vi "Cryomagnetics Get Controls.vi"(8 "error in (no error)":errorcluster, 10 "Data in":T1 {"Fast rate" format="%.4g"; "Low limit, kG" format="%.3g"; "High limit, kG" format="%.3g"; "Rates, A/s" format="%.4g"}, 11 "VISA resource name":refnum<visa-resource-name>) -> (0 "error out":errorcluster, 2 "Data out":T1 {"Fast rate" format="%.4g"; "Low limit, kG" format="%.3g"; "High limit, kG" format="%.3g"; "Rates, A/s" format="%.4g"}, 3 "VISA Resource Name Out":refnum<visa-resource-name>)   [LabVIEW 2015]
uses:
  Cryomagnetics Control Panel Data.ctl
  Sweep mode.ctl
  GPIB/VISA  Send Receive.vi
panel:
  out "Low limit, kG":dbl format="%.3g"
  out "High limit, kG":dbl format="%.3g"
  out "Fast rate":dbl format="%.4g"
  out "Rates":dbl[](array[numeric]) format="%.4g"
  out "Ranges":dbl[](array[numeric])
  # "Magnet Control"
  # "Magnet Control"
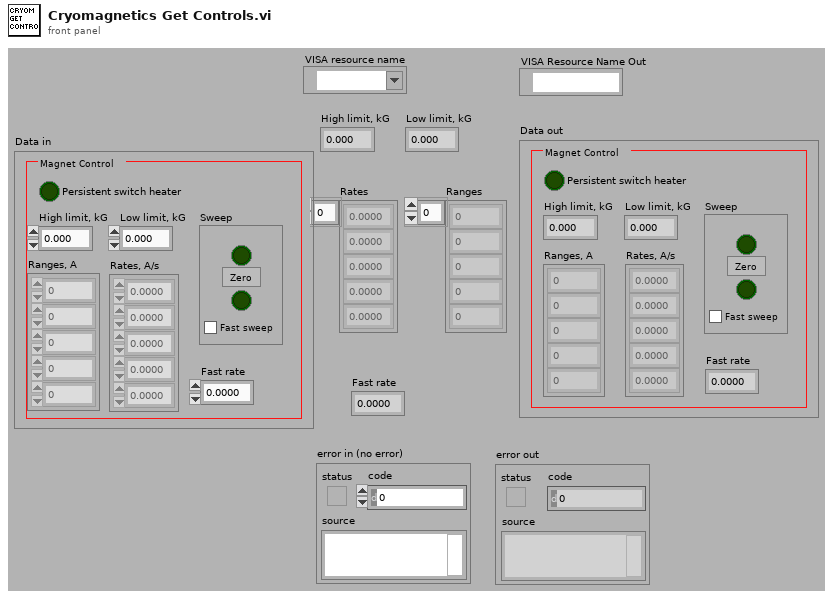
[diagram p1: front panel]
types:
  T1 = typedef "Cryomagnetics Control Panel Data.ctl" = cluster{"Persistent switch heater":bool, "Rates, A/s":dbl[], "Ranges, A":dbl[], "High limit, kG":dbl, "Low limit, kG":dbl, "Sweep ":T2, "Fast rate":dbl}
  T2 = typedef "Sweep mode.ctl" = cluster{"zero":bool, "sweep up":bool, "sweep down":bool, "fast sweep":bool}
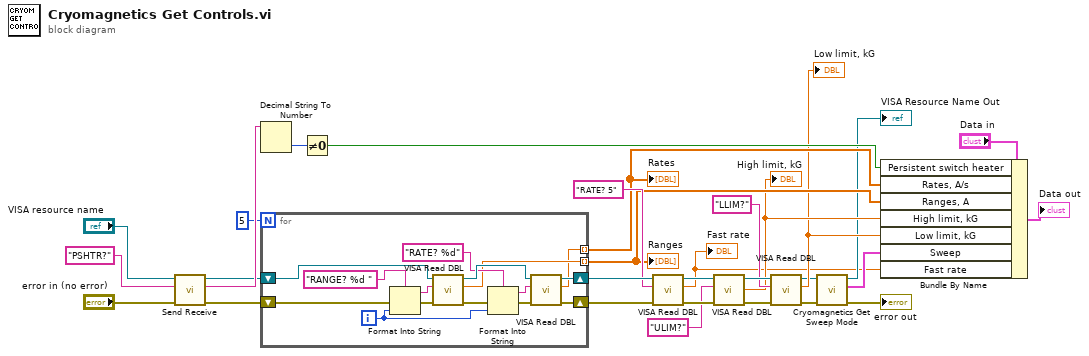
[diagram p0: block diagram]
diagram:
  n1 = call-poly "Send Receive.vi"("error in (no error)"="error in (no error)", "data string in"="PSHTR?", "VISA Resource Name"="VISA resource name") -> ("error out"=w6:errorcluster, "data string out"=w27:string, "VISA Resource Name Out"=w5:refnum<visa-resource-name>)  [unwired: 6 in]
  n2 = Decimal String To Number(string=w27) -> (number=w26:i32)  [unwired: 2 in, 1 out]
  n3 = for {
    N: 5 -> [_]
    shift-right: [w39] -> w23
    shift-left: w5 -> [w45]
    shift-right: [w33] -> w24
    shift-left: w6 -> [w42]
    tunnel: [w32] -> w12 mode=indexing
    tunnel: [w31] -> w13 mode=indexing
    i -> [w37]
    n4 = Format Into String(format string="RANGE? %d ", error in=w42, w37) -> (resulting string=w43:string, error out=w41:errorcluster)  [unwired: 1 in]
    n5 = call "VISA Read DBL.vi"("error in"=w41, "Query string"=w43, "VISA Resource Name"=w45) -> ("error out"=w36:errorcluster, "Value"=w32:dbl, "VISA Resource Name Out"=w40:refnum<visa-resource-name>)  [unwired: 6 in]
    n6 = Format Into String(format string="RATE? %d", error in=w36, w37) -> (resulting string=w34:string, error out=w35:errorcluster)  [unwired: 1 in]
    n7 = call "VISA Read DBL.vi"("error in"=w35, "Query string"=w34, "VISA Resource Name"=w40) -> ("error out"=w33:errorcluster, "Value"=w31:dbl, "VISA Resource Name Out"=w39:refnum<visa-resource-name>)  [unwired: 6 in]
  }
  "Ranges" <- w12
  "Rates" <- w13
  n8 = Not Equal To 0?(x=w26) -> (x != 0?=w14:bool)
  n9 = call "VISA Read DBL.vi"("error in"=w24, "Query string"="RATE? 5" ("data string in"), "VISA Resource Name"=w23) -> ("error out"=w21:errorcluster, "Value"=w2:dbl, "VISA Resource Name Out"=w20:refnum<visa-resource-name>)  [unwired: 6 in]
  "Fast rate" <- w2
  n10 = call "VISA Read DBL.vi"("error in"=w21, "Query string"="ULIM?" ("data string in"), "VISA Resource Name"=w20) -> ("error out"=w18:errorcluster, "Value"=w11:dbl, "VISA Resource Name Out"=w17:refnum<visa-resource-name>)  [unwired: 6 in]
  "High limit, kG" <- w11
  n11 = call "VISA Read DBL.vi"("error in"=w18, "Query string"="LLIM?" ("data string in"), "VISA Resource Name"=w17) -> ("error out"=w9:errorcluster, "Value"=w10:dbl, "VISA Resource Name Out"=w8:refnum<visa-resource-name>)  [unwired: 6 in]
  "Low limit, kG" <- w10
  n12 = call "Cryomagnetics Get Sweep Mode.vi"("error in (no error)"=w9, "VISA Resource Name"=w8) -> ("error out"=→"error out":errorcluster, "sweep mode"=w7:T2, "VISA Resource Name Out"=→"VISA Resource Name Out":refnum<visa-resource-name>)  [unwired: 7 in]
  n13 = Bundle By Name(cluster="Data in", "Persistent switch heater"=w14, "Rates, A/s"=w13, "Ranges, A"=w12, "High limit, kG"=w11, "Low limit, kG"=w10, "Sweep"=w7, "Fast rate"=w2) -> (→"Data out":T1)
